vi "Test Program.vi"() -> ()   [LabVIEW 2018, in "EPOS4.lvlib"]
uses:
  EPOS4.lvlib
  Controls/EPOS Communication Settings.ctl
panel:
  out "axis data":T1
  in  "EPOS4 Settings":T2={"VISA resource name"="", "axis"={"keyHandle"=0, "nodeId"=1}, "Simulated?"=FALSE}
  in  "speed":dbl
  in  "stop":bool
  out "Pump On?":enum16{"Off", "On", "Not Initialized"}(ring)
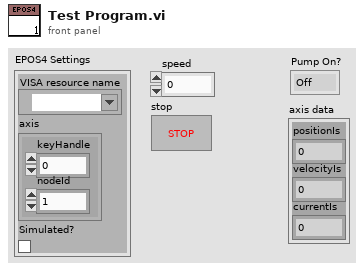
[diagram p1: front panel]
types:
  T1 = cluster{"positionIs":i32, "velocityIs":i32, "currentIs":i16}
  T2 = typedef "EPOS4.lvlib/EPOS Communication Settings.ctl" = cluster{"VISA resource name":refnum<visa-resource-name>, "axis":cluster{"keyHandle":u32, "nodeId":u16}, "Simulated?":bool}
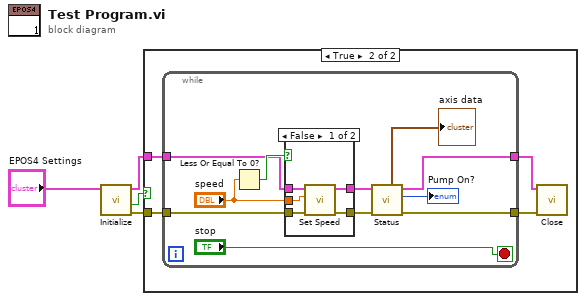
[diagram p0: block diagram]
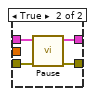
[diagram p3: hidden frame]
diagram:
  n1 = call "Initialize.vi"("EPOS4 Settings In"="EPOS4 Settings") -> ("error out"=w4:errorcluster, "Initialized"=w1:bool, "EPOS4 Settings Out"=w2:T2)  [unwired: 7 in, 1 out]
  n2 = case shown="True" w1 {
    tunnel: w4 -> [_ w8]
    tunnel: w2 -> [_ w6]
    frame False {
    }
    frame True {
      n3 = while {
        tunnel: w6 -> [w11]
        tunnel: [w14] -> w5
        tunnel: w8 -> [w19]
        tunnel: [w12] -> w7
        stop <- "stop" stop-if-true
        n4 = Less Or Equal To 0?(x="speed") -> (x <= 0?=w18:bool)
        n5 = case shown="False" w18 {
          tunnel: [w21 w28] -> w16
          tunnel: w19 -> [w23 w27]
          tunnel: [w22 w26] -> w15
          tunnel: "speed" -> [w24 _]
          tunnel: w11 -> [w20 w25]
          frame False {
            n6 = call "Set Speed.vi"("error in (no error)"=w23, "speed"=w24, "EPOS4 Settings In"=w20) -> ("error out"=w22:errorcluster, "EPOS4 Settings Out"=w21:T2)  [unwired: 6 in, 1 out]
          }
          frame True {
            n7 = call "Pause.vi"("error in (no error)"=w27, "EPOS4 Settings in"=w25) -> ("error out"=w26:errorcluster, "EPOS4 Settings out"=w28:T2)  [unwired: 7 in, 1 out]
          }
        }
        n8 = call "Status.vi"("error in (no error)"=w15, "EPOS4 Settings In"=w16) -> ("error out"=w12:errorcluster, "Centrifuge On?"=→"Pump On?":enum16{"Off", "On", "Not Initialized"}, "EPOS4 Settings Out"=w14:T2, "axis data"=→"axis data":T1)  [unwired: 5 in, 1 out]
      }
      n9 = call "Close.vi"("error in (no error)"=w7, "EPOS4 Settings In"=w5) -> ()  [unwired: 7 in, 3 out]
    }
  }
